vi "Is Empty.vi"(8 "error in (no error)":errorcluster) -> (0 "error out":errorcluster, 3 "Empty?":bool)   [LabVIEW 2020, in "TDS1002 Oscilloscope.lvlib" / "Clone Registration.lvlib"]
doc: "Determine if the cloneable module registry is empty.\n_____\nBased on DQMH Project Template 6.1.0.94.\n____\nPantherLAB Templates 1.0.0.1\nCopyright (c) 2022, PantherLAB\n____\nPantherLAB Templates 1.0.0.5\nCopyright (c) 2022, PantherLAB"
uses:
  Clone Registration.lvlib
  Action--enum.ctl
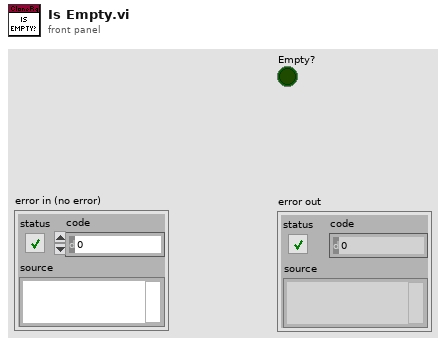
[diagram p1: front panel]
types:
  T1 = typedef "TDS1002 Oscilloscope.lvlib/Clone Registration.lvlib/Action--enum.ctl" = enum16{"Init", "Add Instance", "Remove Instance", "List Instances", "Is First?"}
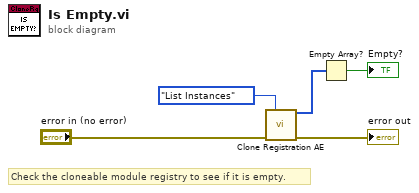
[diagram p0: block diagram]
diagram:
  # "Check the cloneable module registry to see if it is empty."
  n1 = call "Clone Registration AE.vi"("Action"=Action--enum."List Instances", "error in"="error in (no error)") -> ("Module IDs"=w1:i32[], "error out"=→"error out":errorcluster)  [unwired: 5 in, 7 out]
  n2 = Empty Array?(array=w1) -> (empty?=→"Empty?":bool)
